vi "Set Inline (Array).vi"(10 "inline":bool, 11 "Transfer Groups in":refnum<class "Transfer Group.lvclass">[](array[class])) -> (3 "Transfer Groups out":refnum<class "Transfer Group.lvclass">[](array[class]))   [LabVIEW 2021, in "DSF Core.lvlib" / "Transfer Group.lvclass"]
uses:
  Transfer Group.lvclass
  Transfer Group.lvclass/Transfer Group.ctl
  Transfer/Transfer.lvclass/Transfer.ctl
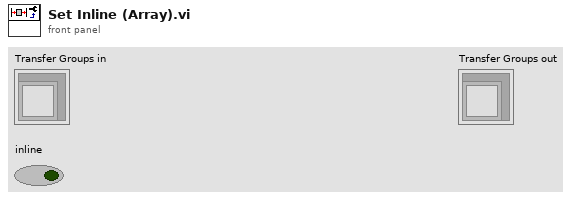
[diagram p1: front panel]
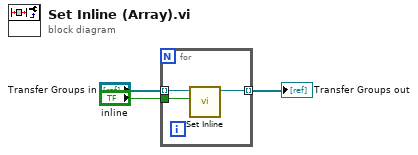
[diagram p0: block diagram]
diagram:
  n1 = for {
    tunnel: "Transfer Groups in" -> [w6] mode=indexing
    tunnel: [w5] -> w2 mode=indexing
    tunnel: "inline" -> [w4]
    n2 = call "Set Inline.vi"("inline"=w4, "Transfer Group in"=w6) -> ("Transfer Group out"=w5:refnum<class "Transfer Group.lvclass">)  [unwired: 9 in]
  }
  "Transfer Groups out" <- w2
